vi "DSF.Shared.Configuration.Framework.Create.vi"(8 "error in (no error)":errorcluster, 11 "configuration path":path) -> (0 "error out":errorcluster, 3 "Framework Configuration":refnum<class "DSF.Shared.Configuration.Framework.lvclass">)   [LabVIEW 2017, in "DSF.Shared.lvlib" / "DSF.Shared.Configuration.Framework.lvclass"]
uses:
  DSF.Shared.Configuration.Framework.lvclass
  DSF.Shared.Configuration.Framework.lvclass/DSF.Shared.Configuration.Framework.ctl
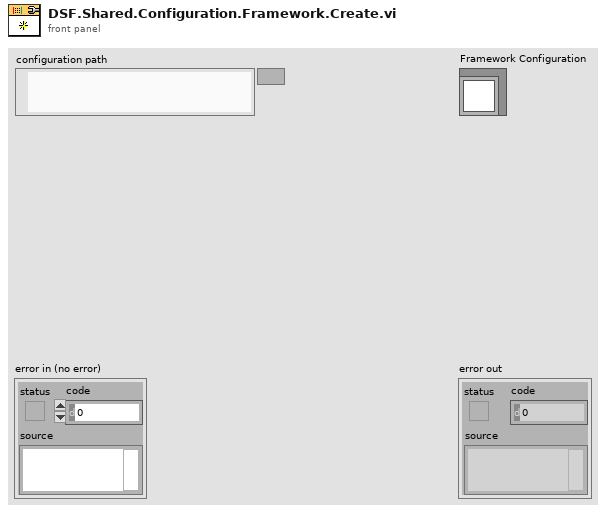
[diagram p1: front panel]
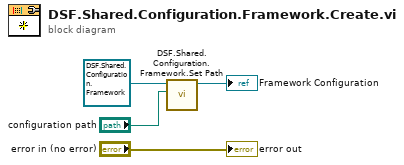
[diagram p0: block diagram]
diagram:
  n1 = call "DSF.Shared.Configuration.Framework.Set Path.vi"("configuration path"="configuration path", "Framework Configuration in"=refnum<class "DSF.Shared.Configuration.Framework.lvclass"> refnum) -> ("Framework Configuration out"=→"Framework Configuration":refnum<class "DSF.Shared.Configuration.Framework.lvclass">)  [unwired: 9 in]
  "error out" <- "error in (no error)"
